vi "Sub_Delete_Fixed_Beam_Location.vi"(11 "Pre-BC Matrix":dbl[][](array[numeric])) -> (3 "Post-BC Matrix":dbl[][](array[numeric]))   [LabVIEW 2021]
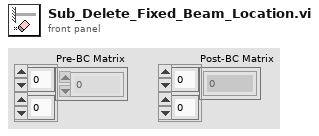
[diagram p1: front panel]
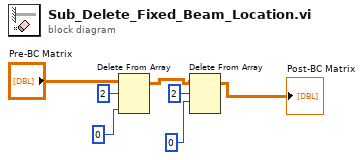
[diagram p0: block diagram]
diagram:
  n1 = Delete From Array(array="Pre-BC Matrix", length=2, index (col)=0 ("disabled index (col)")) -> (array with subset deleted=w2:dbl[][])  [unwired: 1 in, 1 out]
  n2 = Delete From Array(array=w2, length=2, index (row)=0 ("disabled index (col)")) -> (array with subset deleted=→"Post-BC Matrix":dbl[][])  [unwired: 1 in, 1 out]
